vi "Day 1 (Part One).vi"() -> ()   [LabVIEW 2021]
uses:
  7385093b-823c-42d4-ac89-861aca289567.vi
  <vilib>/Comparison/Less/Less Functor/Less Functor.lvclass
panel:
  out "Unique Sum?":bool
  out "Maximum Value":u32
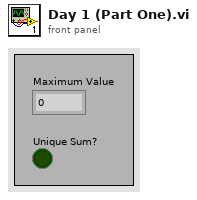
[diagram p1: front panel]
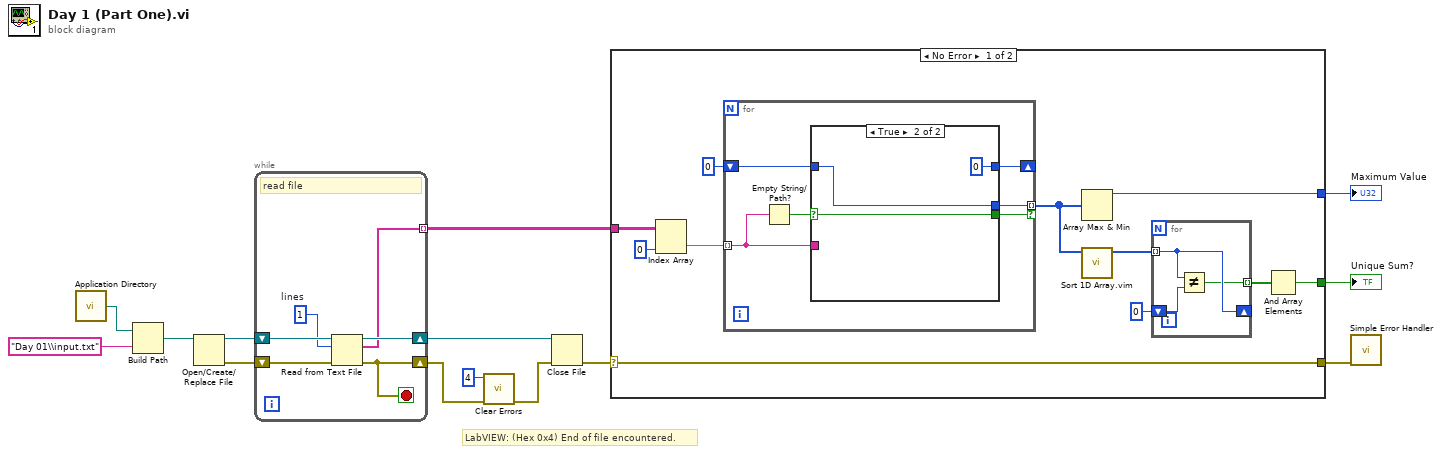
[diagram p0: block diagram]
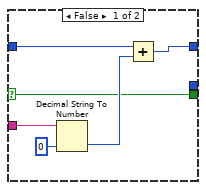
[diagram p2: hidden frame]
diagram:
  # "LabVIEW: (Hex 0x4) End of file encountered."
  n1 = call <vilib>:"Application Directory.vi"() -> ("Application Directory"=w14:path)
  n2 = Build Path(base path=w14, name or relative path="Day 01\\input.txt") -> (appended path=w12:path)
  n3 = Open/Create/Replace File(file path (use dialog)=w12) -> (refnum out=w10:refnum<file>, error out=w11:errorcluster)  [unwired: 5 in, 1 out]
  n4 = while {
    shift-right: [w15] -> w8
    shift-left: w11 -> [w20]
    shift-right: [w18] -> w9
    shift-left: w10 -> [w19]
    tunnel: [w16] -> w5 mode=indexing
    stop <- w15 stop-if-true
    w17 = 1  # lines
    # "read file"
    n5 = Read from Text File(file (use dialog)=w19, count=w17, error in=w20) -> (refnum out=w18:refnum<file>, text=w16:string[], error out=w15:errorcluster)  [unwired: 1 in, 1 out]
  }
  n6 = call <vilib>:"Clear Errors.vi"("error in (no error)"=w8, "specific error code to clear (0: all)"=4) -> ("error out"=w6:errorcluster)  [unwired: 4 in, 1 out]
  n7 = Close File(refnum=w9, error in=w6) -> (error out=w4:errorcluster)  [unwired: 1 out]
  n8 = case shown="No Error" w4 {
    selector: w4 -> [w21 w50]
    tunnel: w5 -> [w31 _]
    tunnel: [w23 _] -> w3
    tunnel: [w22 _] -> w2
    tunnel: [w21 w50] -> w1
    frame No Error {
      n9 = Index Array(array=w31, index (col)=0 ("disabled index (col)")) -> (element=w29:string[])  [unwired: 1 in]
      n10 = for {
        tunnel: w29 -> [w39] mode=indexing
        shift-right: [w37] -> _
        shift-left: u32 0 -> [w38]
        tunnel: [w36] -> w27 mode=indexing if=w35
        n11 = Empty String/Path?(string/path=w39) -> (empty?=w40:bool)
        n12 = case shown="True" w40 {
          selector: w40 -> [w41 w47]
          tunnel: w39 -> [w46 _]
          tunnel: w38 -> [w43 w48]
          tunnel: [w42 u32 0] -> w37
          tunnel: [_ w48] -> w36
          tunnel: [w41 w47] -> w35
          frame False {
            n13 = Decimal String To Number(string=w46, default (0L)=u32 0 ("default (0 I32)")) -> (number=w44:u32)  [unwired: 1 in, 1 out]
            n14 = Add(x=w43, y=w44) -> (x+y=w42:u32)
          }
          frame True {
          }
        }
      }
      n15 = Array Max & Min(array=w27) -> (max value=w23:u32)  [unwired: 3 out]
      n16 = call "Sort 1D Array.vim"("unsorted array"=w27) -> ("sorted array"=w26:u32[])  [unwired: 10 in]
      n17 = for {
        tunnel: w26 -> [w34] mode=indexing
        shift-right: [w34] -> _
        shift-left: u32 0 -> [w33]
        tunnel: [w32] -> w24 mode=indexing
        n18 = Not Equal?(x=w34, y=w33) -> (x != y?=w32:bool)
      }
      n19 = And Array Elements(Boolean array=w24) -> (logical AND=w22:bool)
    }
    frame Error {
    }
  }
  "Maximum Value" <- w3
  "Unique Sum?" <- w2
  n20 = call <vilib>:"Simple Error Handler.vi"("error in (no error)"=w1) -> ()  [unwired: 4 in, 5 out]
